vi "accArray.vi"(11 "data length":i32=4096) -> (3 "Array":dbl[](array[numeric]))   [LabVIEW 2015]
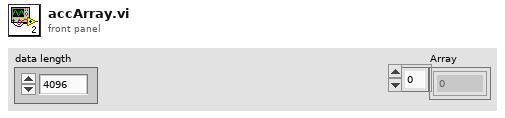
[diagram p1: front panel]
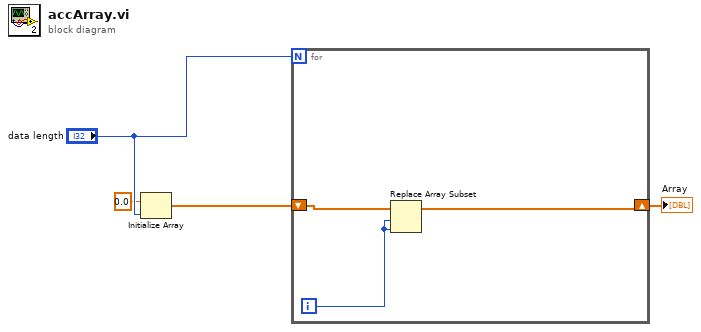
[diagram p0: block diagram]
diagram:
  n1 = Initialize Array(0.0 ("element"), "data length") -> (w2:dbl[])
  n2 = for {
    N: "data length" -> [_]
    shift-right: [w6] -> w1
    shift-left: w2 -> [w7]
    i -> [w5]
    n3 = Replace Array Subset(array=w7, new element=w5, index=w5) -> (w6:dbl[])
  }
  "Array" <- w1
